vi "Global - IP Address.vi"() -> ()   [LabVIEW 2019]
panel:
  in  "IP":string[](array[string])
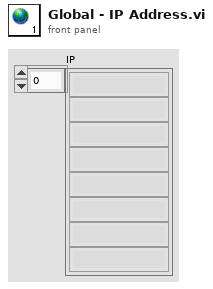
[diagram p1: front panel]
diagram:
